vi "Unflatten.vi"(8 "error in (no error)":errorcluster, 11 "Function Gen Scan in":refnum<class "Function Gen Scan.lvclass">) -> (0 "error out":errorcluster, 3 "Function Gen Scan out":refnum<class "Function Gen Scan.lvclass">)   [LabVIEW 2009, in "Function Gen Scan.lvclass"]
uses:
  Function Gen Scan.lvclass
  Scanner/Scanner.lvclass
  Global/File Locations.vi
  Function Gen Scan.lvclass/Function Gen Scan.ctl
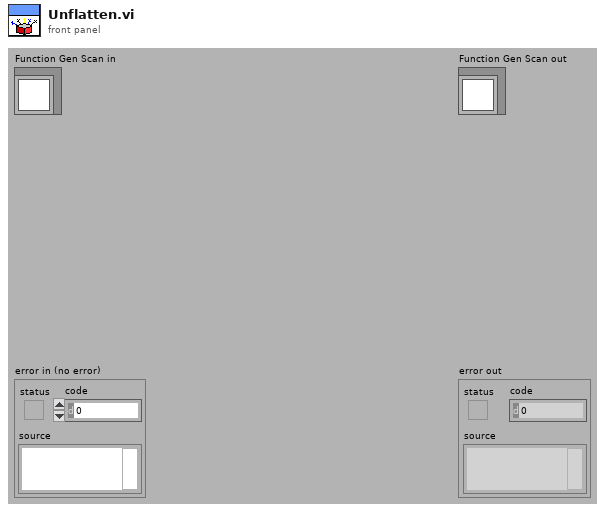
[diagram p1: front panel]
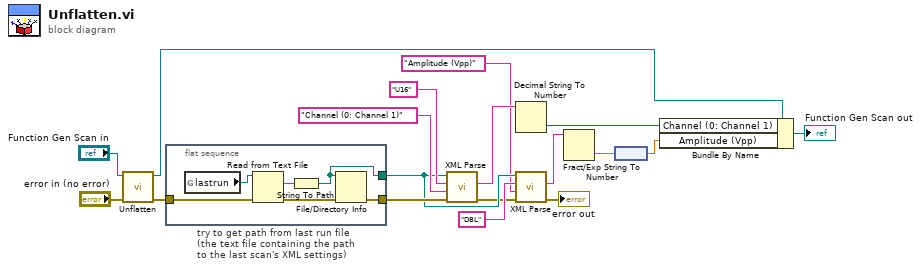
[diagram p0: block diagram]
diagram:
  n1 = call-parent "Unflatten.vi"("error in (no error)"="error in (no error)", "Scanner in"="Function Gen Scan in") -> ("error out"=w15:errorcluster, "Scanner out"=w18:refnum<class "Function Gen Scan.lvclass">)  [unwired: 8 in]
  n2 = flat-sequence "try to get path from last run file\n(the text file containing the path\nto the last scan's XML settings)" {
    tunnel: [w24] -> w7
    tunnel: [w20] -> w13
    tunnel: w15 -> [w19]
    frame #0 {
      n3 = global read "File Locations.vi" "lastrun"() -> (w22:path)
      n4 = Read from Text File(file (use dialog)=w22, error in=w19) -> (text=w23:string, error out=w21:errorcluster)  [unwired: 4 out]
      n5 = String To Path(string=w23) -> (path=w24:path)
      n6 = File/Directory Info(path=w24, error in=w21) -> (error out=w20:errorcluster)  [unwired: 6 out]
    }
  }
  n7 = call "XML Parse.vi"("error in (no error)"=w13, "Name String"="Channel (0: Channel 1)", "Type String"="U16", "Path"=w7) -> ("error out"=w5:errorcluster, "String Out"=w10:string)  [unwired: 6 in]
  n8 = Decimal String To Number(string=w10) -> (number=w9:i32)  [unwired: 2 in, 1 out]
  n9 = call "XML Parse.vi"("error in (no error)"=w5, "Name String"="Amplitude (Vpp)", "Type String"="DBL", "Path"=w7) -> ("error out"=→"error out":errorcluster, "String Out"=w3:string)  [unwired: 6 in]
  n10 = Fract/Exp String To Number(string=w3) -> (number=w4:dbl)  [unwired: 3 in, 1 out]
  n11 = node(w4) -> (w2:dbl[unit])
  n12 = Bundle By Name(cluster=w18, "Channel (0: Channel 1)"=w9, "Amplitude (Vpp)"=w2) -> (→"Function Gen Scan out":refnum<class "Function Gen Scan.lvclass">)
